vi "TalkPort.vi"(6 "IsEnabled":bool, 7 "error constant":errorcluster, 8 "StopThread":bool, 9 "OutString":string, 10 "Port":u16) -> (0 "error out":errorcluster, 1 "Socket Closed":bool)   [LabVIEW 2019]
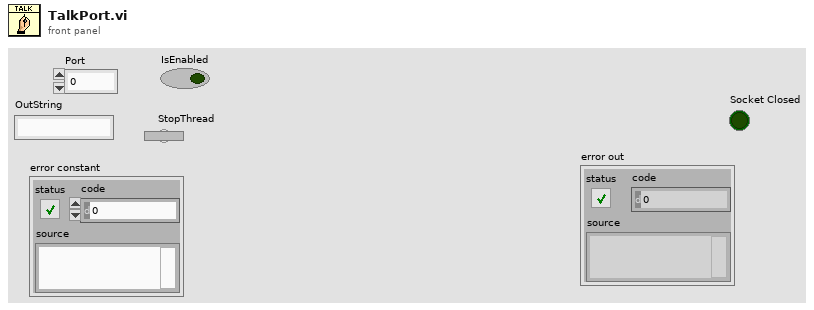
[diagram p1: front panel]
types:
  T1 = enum16{"Standard", "Buffered", "CRLF", "Immediate"}
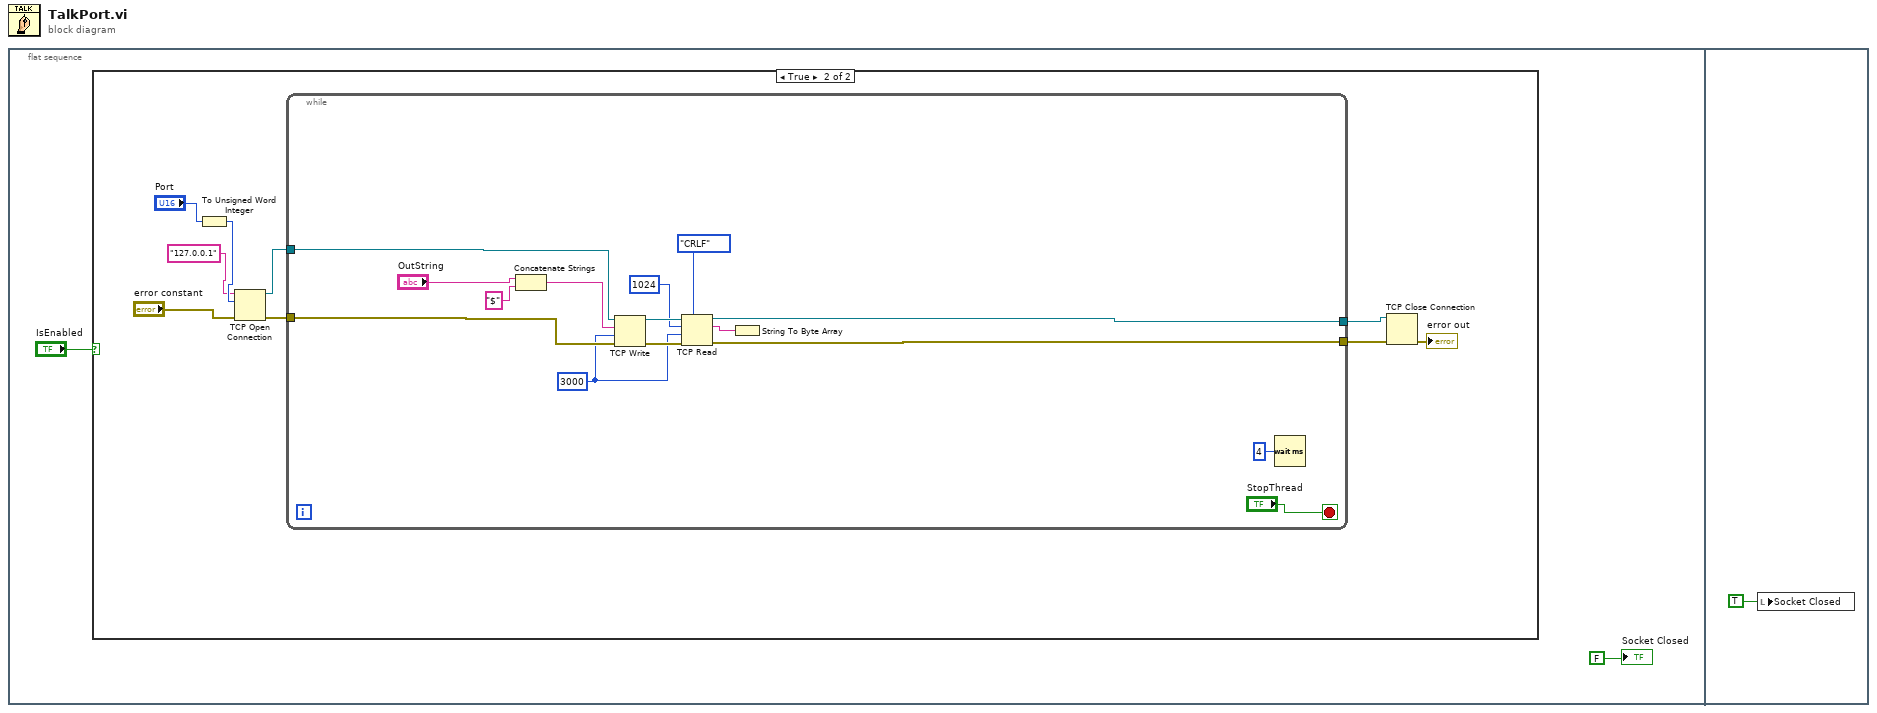
[diagram p0: block diagram]
diagram:
  n1 = flat-sequence {
    frame #0 {
      n2 = case shown="True" "IsEnabled" {
        frame False {
        }
        frame True {
          n3 = To Unsigned Word Integer(number="Port") -> (unsigned 16bit integer=w5:u16)
          n4 = TCP Open Connection(address="127.0.0.1", remote port or service name=w5, error in (no error)="error constant") -> (connection ID=w9:refnum<k5>, error out=w7:errorcluster)  [unwired: 2 in]
          n5 = while {
            tunnel: w7 -> [w25]
            tunnel: [w17] -> w8
            tunnel: w9 -> [w23]
            tunnel: [w16] -> w10
            stop <- "StopThread" stop-if-true
            w20 = 3000 ("timeout ms (25000)")
            n6 = Concatenate Strings("OutString", "$" ("string")) -> (w14:string)
            n7 = TCP Write(connection ID=w23, data in=w14, error in (no error)=w25, 9:w20) -> (connection ID out=w21:refnum<k5>, error out=w22:errorcluster)  [unwired: 1 out]
            n8 = TCP Read(connection ID=w21, bytes to read=1024, error in (no error)=w22, 7:T1."CRLF" ("mode (standard)"), 9:w20) -> (connection ID out=w16:refnum<k5>, data out=w18:string, error out=w17:errorcluster)
            n9 = String To Byte Array(string=w18) -> ()  [unwired: 1 out]
            n10 = Wait (ms)(milliseconds to wait=u32 4) -> ()  [unwired: 1 out]
          }
          n11 = TCP Close Connection(connection ID=w10, error in (no error)=w8) -> (error out=→"error out":errorcluster)  [unwired: 1 in, 1 out]
        }
      }
      "Socket Closed" <- FALSE
    }
    frame #1 {
      n12 = local write "Socket Closed"(TRUE) -> ()
    }
  }
